vi "ChipKit BlinkM.vi"() -> ()   [LabVIEW 2011, in "LabVIEW Interface for ChipKit.lvlib"]
doc: "An example that uses I2C to control a BlinkM."
uses:
  vi.lib/LabVIEW Interface for ChipKit/LabVIEW Interface for ChipKit.lvlib
panel:
  in  "VISA resource name":refnum<visa-resource-name>
  out "Color":u32(colorbox)
  in  "Blue":u8(slide) scale=0.0..255.0
  in  "Green":u8(slide) scale=0.0..255.0
  in  "Stop":bool
  in  "Red":u8(slide) scale=0.0..255.0
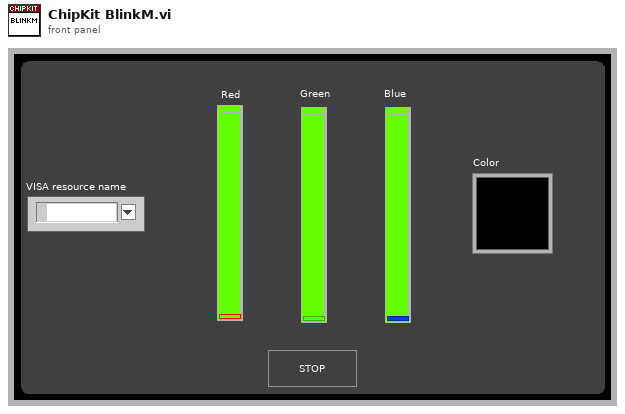
[diagram p1: front panel]
types:
  T1 = typedef "LabVIEW Interface for ChipKit.lvlib/Chipkit Resource.ctl" = cluster{"VISA resource":refnum<visa-resource-name>, "Board Type":T2, "Connection Type":enum8{"USB / Serial"}, "Bytes Per Packet (15)":u8}
  T2 = typedef "LabVIEW Interface for ChipKit.lvlib/Board Type.ctl" = enum16{"Arduino Uno", "Dimuelanove w/Atmega 328", "Mega 2560", "Chipkit Uno32", "Chipkit Max32"}
  T3 = typedef "LabVIEW Interface for ChipKit.lvlib/Chipkit Resource.ctl" = cluster{"COM Port":refnum<visa-resource-name>, "Board Type":T4, "Connection Type":T5, "Baud Rate (115200)":u32, "Bytes Per Packet (15)":u32}
  T4 = typedef "LabVIEW Interface for ChipKit.lvlib/Board Type.ctl" = enum16{"ChipKit uC32", "ChipKit Uno32", "ChipKit Max32"}
  T5 = typedef "LabVIEW Interface for ChipKit.lvlib/Connection Type.ctl" = enum8{"USB / Serial", "XBEE", "BlueSmirf (Bluetooth)"}
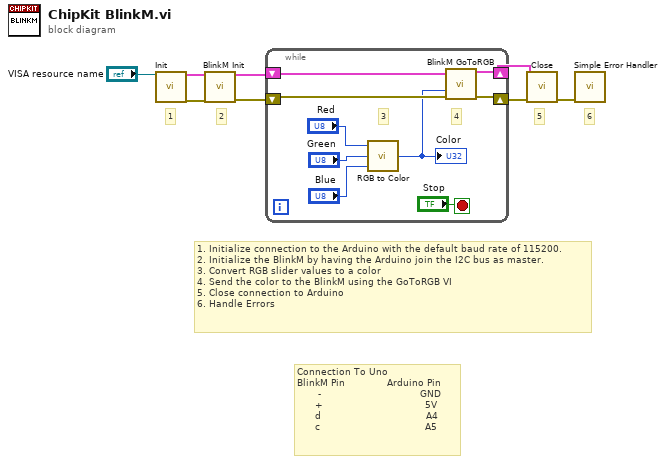
[diagram p0: block diagram]
diagram:
  # "Connection To Uno\nBlinkM Pin              Arduino Pin\n       -                                 GND\n      +                                  5V\n      d                                   A4 \n      c                                   A5"
  # "6"
  # "5"
  # "2"
  # "1"
  # "1. Initialize connection to the Arduino with the default baud rate of 115200.\n2. Initialize the BlinkM by having the Arduino join the I2C bus as master.\n3. Convert RGB slider values to a color\n4. Send the color to the BlinkM using the GoToRGB VI\n5. Close connection to Arduino\n6. Handle Errors"
  n1 = call "Init.vi"("VISA resource"="VISA resource name") -> ("Arduino Resource"=w7:T1, "error out"=w6:errorcluster)  [unwired: 17 in]
  n2 = call "BlinkM Init.vi"("Arduino Resource"=w7, "error in"=w6) -> ("Arduino Resource"=w5:T3, "error out"=w4:errorcluster)  [unwired: 12 in]
  n3 = while {
    shift-right: [w13] -> w3
    shift-left: w5 -> [w9]
    shift-right: [w12] -> w2
    shift-left: w4 -> [w11]
    stop <- "Stop" stop-if-true
    # "3"
    # "4"
    n4 = call <vilib>:"RGB to Color.vi"("B"="Blue", "G"="Green", "R"="Red") -> ("Color"=w10:u32)
    "Color" <- w10
    n5 = call "BlinkM GoToRGB.vi"("Arduino Resource"=w9, "Color"=w10, "error in"=w11) -> ("Arduino Resource"=w13:T3, "error out"=w12:errorcluster)  [unwired: 11 in]
  }
  n6 = call "Close.vi"("Arduino Resource"=w3, "error in"=w2) -> ("error out"=w8:errorcluster)  [unwired: 13 in]
  n7 = call <vilib>:"Simple Error Handler.vi"("error in (no error)"=w8) -> ()  [unwired: 4 in, 5 out]
